vi "Periodic Tasks.vi"(7 "Chassis X SPD":dbl=0.7, 8 "error in":errorcluster) -> ()   [LabVIEW 2019]
doc: "This VI runs in parallel to other tasks. It can contain as many user-defined periodic loops as you need. These can carry out PID or other sorts of timed response."
uses:
  <vilib>/Rock Robotics/WPI/Utilities/WPI_GetSetVariantRefNum.vi
  Robot Global Data.vi
  <vilib>/Rock Robotics/Network Tables/NT Read Number.vi
  <vilib>/Rock Robotics/WPI/RobotDrive/WPI_RobotDriveArcadeDrive_Standard(NoSaturation).vi
  <vilib>/Rock Robotics/Network Tables/NT Read Boolean.vi
  <vilib>/Rock Robotics/Network Tables/NT Write Number.vi
panel:
  in  "Chassis Y SPD":dbl=0.7
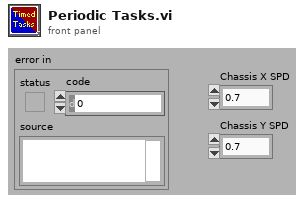
[diagram p1: front panel]
types:
  T1 = typedef "WPI_JoystickDevRef.ctl" = cluster{"Device":T2}
  T2 = typedef "WPI_JoystickDeviceEnum.ctl" = enum16{"USB 0", "USB 1", "USB 2", "USB 3", "USB 4", "USB 5"}
  T3 = typedef "WPI_RobotDriveDevRef.ctl" = cluster{"DevStatus":errorcluster, "Motors[]":T4[], "Square Inputs":bool, "Max Output":dbl}
  T4 = typedef "WPI_MotorControlDeviceRef.ctl" = cluster{"DeviceStatus":errorcluster, "Type":T5, "PWM":cluster{"PWM Channel":T6, "DeadBand":T7}, "CAN":cluster{"Device Number":u8, "SetOutput VI Ref":variant, "GetOutput VI Ref":variant, "Enable VI Ref":variant, "Disable VI Ref":variant, "Data":variant}, "Invert":bool, "DIO PWM":cluster{"PWM \"Enable\" Channel":T6, "DIOChannel":T8, "PWM Rate":dbl}}
  T5 = typedef "WPI_MotorControlType.ctl" = enum16{"PWM", "CAN", "DIO PWM"}
  T6 = typedef "FPGA_DIOPWMChannel.ctl" = enum8{"PWM 0", "PWM 1", "PWM 2", "PWM 3", "PWM 4", "PWM 5", "PWM 6", "PWM 7", "PWM 8", "PWM 9", "PWM MXP 0", "PWM MXP 1", "PWM MXP 2", "PWM MXP 3", "PWM MXP 4", "PWM MXP 5", "PWM MXP 6", "PWM MXP 7", "PWM MXP 8", "PWM MXP 9", "Invalid"}
  T7 = typedef "WPI_PWMDeadband.ctl" = cluster{"Name":string, "maxPositivePwm":i32, "minPositivePwm":i32, "centerPwm":i32, "maxNegativePwm":i32, "minNegativePwm":i32, "angularRange":u16}
  T8 = typedef "FPGA_DIOChannel.ctl" = enum8{"DIO 0", "DIO 1", "DIO 2", "DIO 3", "DIO 4", "DIO 5", "DIO 6", "DIO 7", "DIO 8", "DIO 9", "DIO MXP 0", "DIO MXP 1", "DIO MXP 2", "DIO MXP 3", "DIO MXP 4", "DIO MXP 5", "DIO MXP 6", "DIO MXP 7", "DIO MXP 8", "DIO MXP 9", "DIO MXP 10", "DIO MXP 11", "DIO MXP 12", "DIO MXP 13", "DIO MXP 14", "DIO MXP 15", "SPI Port CS1", "SPI Port CS2", "SPI Port CS3", "SPI Port MISO", "SPI Port MOSI", "Invalid"}
  T9 = cluster{"JoystickDevRef":T1, "RobotDriveDevRef":T3}
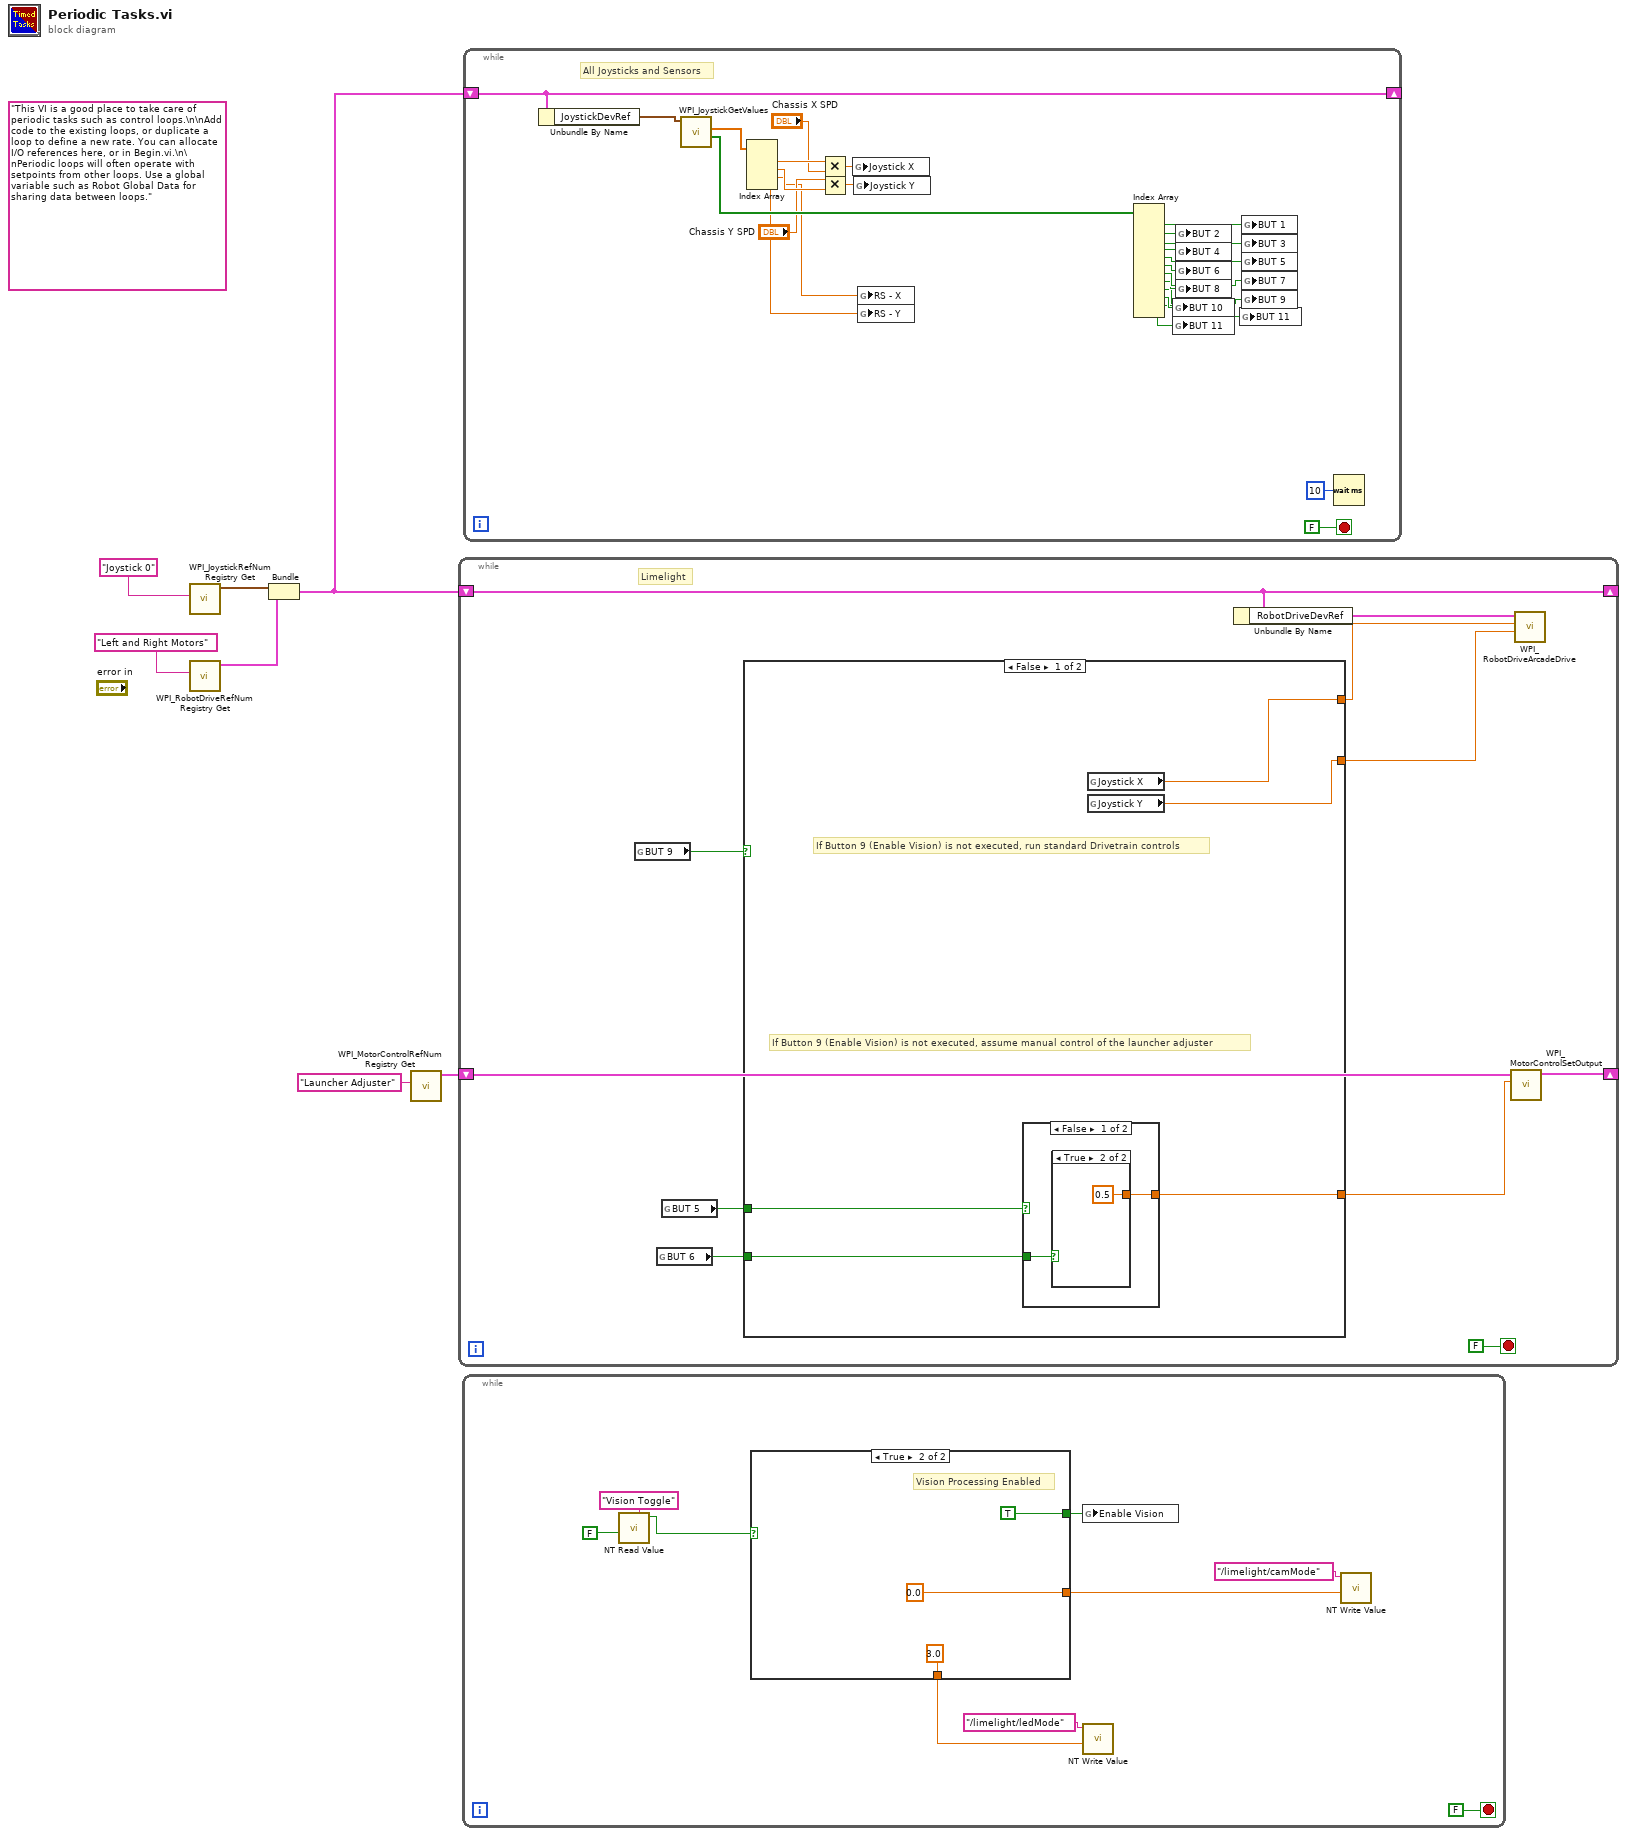
[diagram p0: block diagram]
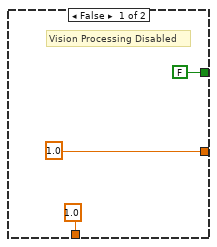
[diagram p2: hidden frame]
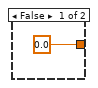
[diagram p3: hidden frame]
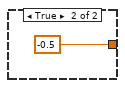
[diagram p4: hidden frame]
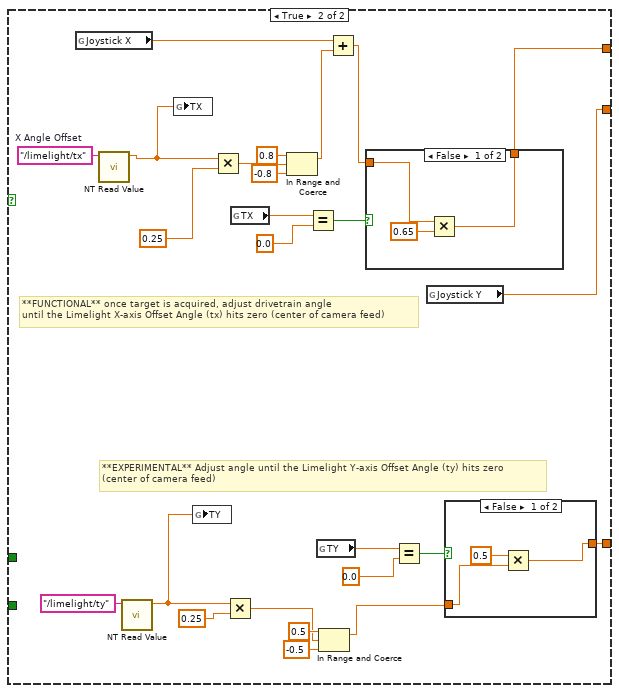
[diagram p5: hidden frame]
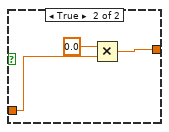
[diagram p6: hidden frame]
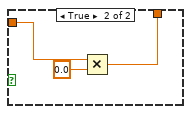
[diagram p7: hidden frame]
diagram:
  (unwired) "This VI is a good place to take care of periodic tasks such as control loops.\n\nAdd code to the existing loops, or duplicate a loop to define a new rate. You can allocate I/O references here, or in Begin.vi.\n\nPeriodic loops will often operate with setpoints from other loops. Use a global variable such as Robot Global Data for sharing data between loops."
  n1 = call <vilib>:"WPI_JoystickRefNum Registry Get.vi"("refnum name"="Joystick 0") -> ("JoystickDevRef"=w5:T1)  [unwired: 1 in, 9 out]
  n2 = call <vilib>:"WPI_RobotDriveRefNum Registry Get.vi"("refnum name"="Left and Right Motors") -> ("RobotDriveDevRef"=w4:T3)  [unwired: 1 in, 9 out]
  n3 = Bundle("JoystickDevRef"=w5, "RobotDriveDevRef"=w4) -> (w3:T9)  [unwired: 1 out]
  n4 = call <vilib>:"WPI_MotorControlRefNum Registry Get.vi"("refnum name"="Launcher Adjuster") -> ("MotorControlDevRef"=w2:T4)  [unwired: 9 in, 1 out]
  n5 = while {
    shift-right: [w17] -> _
    shift-left: w3 -> [w17]
    shift-right: [w12] -> _
    shift-left: w2 -> [w11]
    stop <- FALSE stop-if-true
    # "Limelight"
    n6 = global read "Robot Global Data.vi" "BUT 9"() -> (w16:bool)
    n7 = global read "Robot Global Data.vi" "BUT 6"() -> (w8:bool)
    n8 = global read "Robot Global Data.vi" "BUT 5"() -> (w9:bool)
    n9 = case shown="False" w16 {
      tunnel: [w23 w44] -> w14
      tunnel: [w22 w40] -> w13
      tunnel: [w21 w33] -> w10
      tunnel: w9 -> [w20 _]
      tunnel: w8 -> [w19 _]
      frame False {
        # "If Button 9 (Enable Vision) is not executed, assume manual control of the launcher adjuster"
        # "If Button 9 (Enable Vision) is not executed, run standard Drivetrain controls"
        n10 = case shown="False" w20 {
          tunnel: [w25 -0.5] -> w21
          tunnel: w19 -> [w24 _]
          frame False {
            n11 = case shown="True" w24 {
              tunnel: [0.0 0.5] -> w25
              frame False {
              }
              frame True {
              }
            }
          }
          frame True {
          }
        }
        n12 = global read "Robot Global Data.vi" "Joystick X"() -> (w23:dbl)
        n13 = global read "Robot Global Data.vi" "Joystick Y"() -> (w22:dbl)
      }
      frame True {
        w53 = "/limelight/tx"  # X Angle Offset
        # "**FUNCTIONAL** once target is acquired, adjust drivetrain angle \nuntil the Limelight X-axis Offset Angle (tx) hits zero (center of camera feed)"
        # "**EXPERIMENTAL** Adjust angle until the Limelight Y-axis Offset Angle (ty) hits zero\n(center of camera feed)"
        n14 = global read "Robot Global Data.vi" "Joystick X"() -> (w52:dbl)
        n15 = call-poly <vilib>:"NT Read Value.vi"("Name"=w53) -> ("Numeric"=w46:dbl)  [unwired: 9 in, 1 out]
        n16 = call-poly <vilib>:"NT Read Value.vi"("Name"="/limelight/ty") -> ("Numeric"=w38:dbl)  [unwired: 9 in, 1 out]
        n17 = global write "Robot Global Data.vi" "TX"(w46) -> ()
        n18 = global write "Robot Global Data.vi" "TY"(w38) -> ()
        n19 = Multiply(x=w46, y=0.25) -> (x*y=w50:dbl)
        n20 = Multiply(x=w38, y=0.25) -> (x*y=w30:dbl)
        n21 = global read "Robot Global Data.vi" "TX"() -> (w42:dbl)
        n22 = In Range and Coerce(upper limit=0.8, x=w50, lower limit=-0.8) -> (coerced(x)=w51:dbl)  [unwired: 1 out]
        n23 = Equal?(x=w42, y=0.0) -> (x = y?=w43:bool)
        n24 = global read "Robot Global Data.vi" "TY"() -> (w36:dbl)
        n25 = In Range and Coerce(upper limit=0.5, x=w30, lower limit=-0.5) -> (coerced(x)=w29:dbl)  [unwired: 1 out]
        n26 = Add(x=w52, y=w51) -> (x+y=w45:dbl)
        n27 = case shown="False" w43 {
          tunnel: w45 -> [w61 w65]
          tunnel: [w62 w63] -> w44
          frame False {
            n28 = Multiply(x=w61, y=0.65) -> (x*y=w62:dbl)
          }
          frame True {
            n29 = Multiply(x=w65, y=0.0) -> (x*y=w63:dbl)
          }
        }
        n30 = Equal?(x=w36, y=0.0) -> (x = y?=w34:bool)
        n31 = global read "Robot Global Data.vi" "Joystick Y"() -> (w40:dbl)
        n32 = case shown="False" w34 {
          tunnel: [w54 w59] -> w33
          tunnel: w29 -> [w56 w58]
          frame False {
            n33 = Multiply(x=0.5, y=w56) -> (x*y=w54:dbl)
          }
          frame True {
            n34 = Multiply(x=0.0, y=w58) -> (x*y=w59:dbl)
          }
        }
      }
    }
    n35 = Unbundle By Name(w17) -> ("RobotDriveDevRef"=w15:T3)
    n36 = call <vilib>:"WPI_MotorControlSetOutput.vi"("Output"=w10, "MotorControlDevRef"=w11) -> ("MotorControlDevRef"=w12:T4)  [unwired: 7 in, 2 out]
    n37 = call-poly <vilib>:"WPI_RobotDriveArcadeDrive.vi"("Y axis value"=w13, "X axis value"=w14, "RobotDriveDevRef"=w15) -> ()  [unwired: 6 in, 3 out]
  }
  n38 = while {
    stop <- FALSE stop-if-true
    n39 = call-poly <vilib>:"NT Read Value.vi"("Default Value"=FALSE, "Name"="Vision Toggle") -> ("Boolean"=w74:bool)  [unwired: 8 in, 1 out]
    n40 = case shown="True" w74 {
      tunnel: [FALSE ("Enable Vision") TRUE ("Enable Vision")] -> w71
      tunnel: [1.0 ("Numeric") 0.0 ("Numeric")] -> w72
      tunnel: [1.0 ("Numeric") 3.0 ("Numeric")] -> w73
      frame False {
        # "Vision Processing Disabled"
      }
      frame True {
        # "Vision Processing Enabled"
      }
    }
    n41 = global write "Robot Global Data.vi" "Enable Vision"(w71) -> ()
    n42 = call-poly <vilib>:"NT Write Value.vi"("Numeric"=w73, "Name"="/limelight/ledMode") -> ()  [unwired: 9 in, 1 out]
    n43 = call-poly <vilib>:"NT Write Value.vi"("Numeric"=w72, "Name"="/limelight/camMode") -> ()  [unwired: 9 in, 1 out]
  }
  n44 = while {
    shift-right: [w90] -> _
    shift-left: w3 -> [w90]
    stop <- FALSE stop-if-true
    # "All Joysticks and Sensors"
    n45 = Unbundle By Name(w90) -> ("JoystickDevRef"=w104:T1)
    n46 = call <vilib>:"WPI_JoystickGetValues.vi"("JoystickDevRef"=w104) -> ("Buttons"=w103:bool[], "Axes"=w89:dbl[])  [unwired: 6 in, 3 out]
    n47 = Index Array(array=w89) -> (element #1=w86:dbl, element #2=w85:dbl, element #3=w82:dbl, element #4=w81:dbl)  [unwired: 4 in]
    n48 = Multiply(x=w86, y="Chassis X SPD") -> (x*y=w88:dbl)
    n49 = Multiply(x="Chassis Y SPD", y=w85) -> (x*y=w87:dbl)
    n50 = global write "Robot Global Data.vi" "Joystick X"(w88) -> ()
    n51 = global write "Robot Global Data.vi" "Joystick Y"(w87) -> ()
    n52 = global write "Robot Global Data.vi" "RS - X"(w82) -> ()
    n53 = global write "Robot Global Data.vi" "RS - Y"(w81) -> ()
    n54 = Index Array(array=w103) -> (element #1=w102:bool, element #2=w101:bool, element #3=w100:bool, element #4=w99:bool, element #5=w98:bool, element #6=w97:bool, element #7=w96:bool, element #8=w95:bool, element #9=w94:bool, element #10=w93:bool, element #11=w92:bool, element #12=w91:bool)  [unwired: 12 in]
    n55 = global write "Robot Global Data.vi" "BUT 10"(w93) -> ()
    n56 = global write "Robot Global Data.vi" "BUT 11"(w91) -> ()
    n57 = global write "Robot Global Data.vi" "BUT 2"(w101) -> ()
    n58 = global write "Robot Global Data.vi" "BUT 4"(w99) -> ()
    n59 = global write "Robot Global Data.vi" "BUT 6"(w97) -> ()
    n60 = global write "Robot Global Data.vi" "BUT 8"(w95) -> ()
    n61 = global write "Robot Global Data.vi" "BUT 11"(w92) -> ()
    n62 = global write "Robot Global Data.vi" "BUT 1"(w102) -> ()
    n63 = global write "Robot Global Data.vi" "BUT 3"(w100) -> ()
    n64 = global write "Robot Global Data.vi" "BUT 5"(w98) -> ()
    n65 = global write "Robot Global Data.vi" "BUT 7"(w96) -> ()
    n66 = global write "Robot Global Data.vi" "BUT 9"(w94) -> ()
    n67 = Wait (ms)(milliseconds to wait=u32 10) -> ()  [unwired: 1 out]
  }
